vi "ECS - XNET Control Parameters.vi"(8 "XNET Control Parameters":T1, 11 "Rx Data":dbl format="%.2f") -> ()   [LabVIEW 2015, in "ECS-RT.lvlib"]
uses:
  ECS-RT.lvlib
  Typedefs/MISC/Control Parameters.ctl
  Globals/NOx Global.vi
  ECS-Shared.lvlib
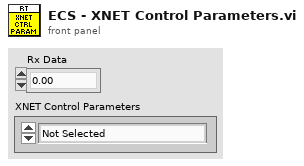
[diagram p1: front panel]
types:
  T1 = typedef "ECS-Shared.lvlib/Control Parameters.ctl" = enum16{"Not Selected", "Pedal Position [%]", "ESTOP", "Sensor1NOx", "Sensor1O2", "Sensor1SupplyStatus", "Sensor1TempStatus", "Sensor1NOxStatus", "Sensor1O2Status", "Sensor1HeaterMode", "Sensor1HeaterCircuit", "Sensor1NOxCircuit", "Sensor1O2Circuit", "Sensor2NOx", "Sensor2O2", "Sensor2SupplyStatus", "Sensor2TempStatus", "Sensor2NOxStatus", "Sensor2O2Status", "Sensor2HeaterMode", "Sensor2HeaterCircuit", "Sensor2NOxCircuit", "Sensor2O2Circuit"}
  T2 = cluster{"NOx (ppm)":i16, "O2 (%)":sgl, "Sensor Supply Status":u8, "Sensor Temperature Status":u8, "NOx Signal Status":u8, "O2 Signal Status":u8, "Heater Mode Status":u8, "Heater Circuit Status":u8, "NOx Circuit Status":u8, "O2 Circuit Status":u8, "NOx Sensor Module Present":bool}
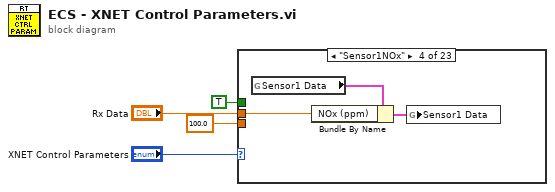
[diagram p0: block diagram]
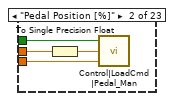
[diagram p3: hidden frame]
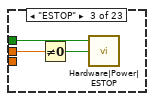
[diagram p4: hidden frame]
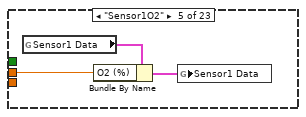
[diagram p5: hidden frame]
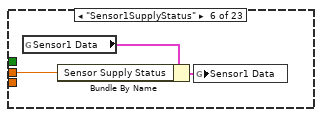
[diagram p6: hidden frame]
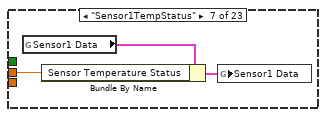
[diagram p7: hidden frame]
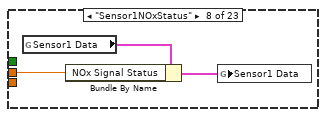
[diagram p8: hidden frame]
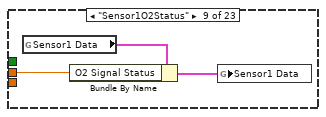
[diagram p9: hidden frame]
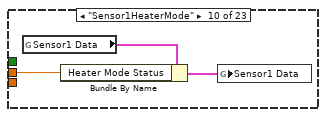
[diagram p10: hidden frame]
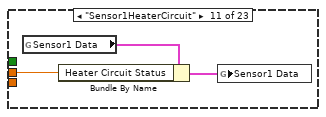
[diagram p11: hidden frame]
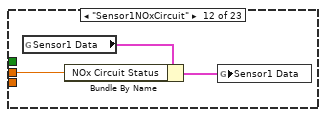
[diagram p12: hidden frame]
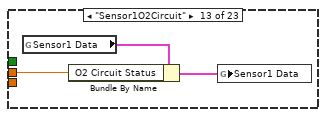
[diagram p13: hidden frame]
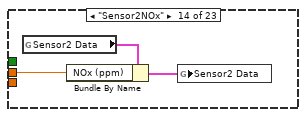
[diagram p14: hidden frame]
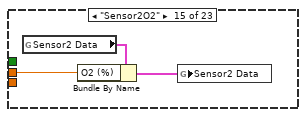
[diagram p15: hidden frame]
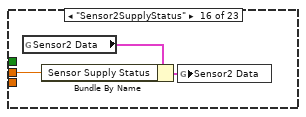
[diagram p16: hidden frame]
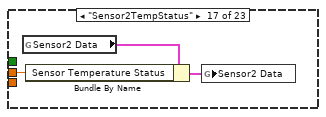
[diagram p17: hidden frame]
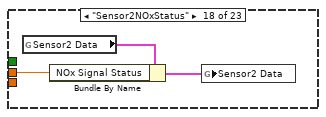
[diagram p18: hidden frame]
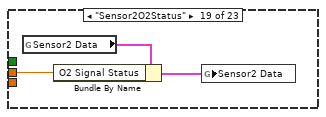
[diagram p19: hidden frame]
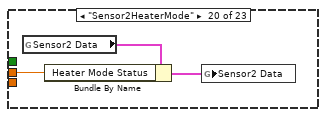
[diagram p20: hidden frame]
diagram:
  n1 = case shown="\"Sensor1NOx\"" "XNET Control Parameters" {
    tunnel: "Rx Data" -> [_ w7 w11 w12 w15 w18 w21 w24 w27 w30 w33 w36 w39 w42 w45 w48 w51 w54 w57 w60 w63 w66 w69]
    tunnel: TRUE ("Adapt") -> [_ w5 w9 _ _ _ _ _ _ _ _ _ _ _ _ _ _ _ _ _ _ _ _]
    tunnel: sgl 100.0 ("%/100") -> [_ w8 _ _ _ _ _ _ _ _ _ _ _ _ _ _ _ _ _ _ _ _ _]
    frame "Not Selected", Default {
    }
    frame "Pedal Position [%]" {
      n2 = To Single Precision Float(number=w7) -> (single precision float=w6:sgl)
      n3 = call "Control|LoadCmd|Pedal_Man"("%/100"=w8, "Value"=w6, "Adapt"=w5) -> ()
    }
    frame "ESTOP" {
      n4 = Not Equal To 0?(x=w11) -> (x != 0?=w10:bool)
      n5 = call "Hardware|Power|ESTOP"("Value"=w10, "Adapt"=w9) -> ()  [unwired: 1 in]
    }
    frame "Sensor1NOx" {
      n6 = global read "NOx Global.vi" "Sensor1 Data"() -> (w14:T2)
      n7 = Bundle By Name(cluster=w14, "NOx (ppm)"=w12) -> (w13:T2)
      n8 = global write "NOx Global.vi" "Sensor1 Data"(w13) -> ()
    }
    frame "Sensor1O2" {
      n9 = global read "NOx Global.vi" "Sensor1 Data"() -> (w17:T2)
      n10 = Bundle By Name(cluster=w17, "O2 (%)"=w15) -> (w16:T2)
      n11 = global write "NOx Global.vi" "Sensor1 Data"(w16) -> ()
    }
    frame "Sensor1SupplyStatus" {
      n12 = global read "NOx Global.vi" "Sensor1 Data"() -> (w20:T2)
      n13 = Bundle By Name(cluster=w20, "Sensor Supply Status"=w18) -> (w19:T2)
      n14 = global write "NOx Global.vi" "Sensor1 Data"(w19) -> ()
    }
    frame "Sensor1TempStatus" {
      n15 = global read "NOx Global.vi" "Sensor1 Data"() -> (w23:T2)
      n16 = Bundle By Name(cluster=w23, "Sensor Temperature Status"=w21) -> (w22:T2)
      n17 = global write "NOx Global.vi" "Sensor1 Data"(w22) -> ()
    }
    frame "Sensor1NOxStatus" {
      n18 = global read "NOx Global.vi" "Sensor1 Data"() -> (w26:T2)
      n19 = Bundle By Name(cluster=w26, "NOx Signal Status"=w24) -> (w25:T2)
      n20 = global write "NOx Global.vi" "Sensor1 Data"(w25) -> ()
    }
    frame "Sensor1O2Status" {
      n21 = global read "NOx Global.vi" "Sensor1 Data"() -> (w29:T2)
      n22 = Bundle By Name(cluster=w29, "O2 Signal Status"=w27) -> (w28:T2)
      n23 = global write "NOx Global.vi" "Sensor1 Data"(w28) -> ()
    }
    frame "Sensor1HeaterMode" {
      n24 = global read "NOx Global.vi" "Sensor1 Data"() -> (w32:T2)
      n25 = Bundle By Name(cluster=w32, "Heater Mode Status"=w30) -> (w31:T2)
      n26 = global write "NOx Global.vi" "Sensor1 Data"(w31) -> ()
    }
    frame "Sensor1HeaterCircuit" {
      n27 = global read "NOx Global.vi" "Sensor1 Data"() -> (w35:T2)
      n28 = Bundle By Name(cluster=w35, "Heater Circuit Status"=w33) -> (w34:T2)
      n29 = global write "NOx Global.vi" "Sensor1 Data"(w34) -> ()
    }
    frame "Sensor1NOxCircuit" {
      n30 = global read "NOx Global.vi" "Sensor1 Data"() -> (w38:T2)
      n31 = Bundle By Name(cluster=w38, "NOx Circuit Status"=w36) -> (w37:T2)
      n32 = global write "NOx Global.vi" "Sensor1 Data"(w37) -> ()
    }
    frame "Sensor1O2Circuit" {
      n33 = global read "NOx Global.vi" "Sensor1 Data"() -> (w41:T2)
      n34 = Bundle By Name(cluster=w41, "O2 Circuit Status"=w39) -> (w40:T2)
      n35 = global write "NOx Global.vi" "Sensor1 Data"(w40) -> ()
    }
    frame "Sensor2NOx" {
      n36 = global read "NOx Global.vi" "Sensor2 Data"() -> (w44:T2)
      n37 = Bundle By Name(cluster=w44, "NOx (ppm)"=w42) -> (w43:T2)
      n38 = global write "NOx Global.vi" "Sensor2 Data"(w43) -> ()
    }
    frame "Sensor2O2" {
      n39 = global read "NOx Global.vi" "Sensor2 Data"() -> (w47:T2)
      n40 = Bundle By Name(cluster=w47, "O2 (%)"=w45) -> (w46:T2)
      n41 = global write "NOx Global.vi" "Sensor2 Data"(w46) -> ()
    }
    frame "Sensor2SupplyStatus" {
      n42 = global read "NOx Global.vi" "Sensor2 Data"() -> (w50:T2)
      n43 = Bundle By Name(cluster=w50, "Sensor Supply Status"=w48) -> (w49:T2)
      n44 = global write "NOx Global.vi" "Sensor2 Data"(w49) -> ()
    }
    frame "Sensor2TempStatus" {
      n45 = global read "NOx Global.vi" "Sensor2 Data"() -> (w53:T2)
      n46 = Bundle By Name(cluster=w53, "Sensor Temperature Status"=w51) -> (w52:T2)
      n47 = global write "NOx Global.vi" "Sensor2 Data"(w52) -> ()
    }
    frame "Sensor2NOxStatus" {
      n48 = global read "NOx Global.vi" "Sensor2 Data"() -> (w56:T2)
      n49 = Bundle By Name(cluster=w56, "NOx Signal Status"=w54) -> (w55:T2)
      n50 = global write "NOx Global.vi" "Sensor2 Data"(w55) -> ()
    }
    frame "Sensor2O2Status" {
      n51 = global read "NOx Global.vi" "Sensor2 Data"() -> (w59:T2)
      n52 = Bundle By Name(cluster=w59, "O2 Signal Status"=w57) -> (w58:T2)
      n53 = global write "NOx Global.vi" "Sensor2 Data"(w58) -> ()
    }
    frame "Sensor2HeaterMode" {
      n54 = global read "NOx Global.vi" "Sensor2 Data"() -> (w62:T2)
      n55 = Bundle By Name(cluster=w62, "Heater Mode Status"=w60) -> (w61:T2)
      n56 = global write "NOx Global.vi" "Sensor2 Data"(w61) -> ()
    }
    frame "Sensor2HeaterCircuit" {
      n57 = global read "NOx Global.vi" "Sensor2 Data"() -> (w65:T2)
      n58 = Bundle By Name(cluster=w65, "Heater Circuit Status"=w63) -> (w64:T2)
      n59 = global write "NOx Global.vi" "Sensor2 Data"(w64) -> ()
    }
    frame "Sensor2NOxCircuit" {
      n60 = global read "NOx Global.vi" "Sensor2 Data"() -> (w68:T2)
      n61 = Bundle By Name(cluster=w68, "NOx Circuit Status"=w66) -> (w67:T2)
      n62 = global write "NOx Global.vi" "Sensor2 Data"(w67) -> ()
    }
    frame "Sensor2O2Circuit" {
      n63 = global read "NOx Global.vi" "Sensor2 Data"() -> (w71:T2)
      n64 = Bundle By Name(cluster=w71, "O2 Circuit Status"=w69) -> (w70:T2)
      n65 = global write "NOx Global.vi" "Sensor2 Data"(w70) -> ()
    }
  }
